vi "Slide Buttons.vi"(8 "error in (no error)":errorcluster, 10 "Distance":i32, 11 "Display State In":T1={"Numeric"=0.0, "Array of Button References"=[], "Space Between Menu Buttons"=0, "Number of Menu Buttons"=0, "Array of Button Names"=[], "Most Recent Vertical Position"=0, "This VI"=refnum, "Current Action"=enum."Not Moving", "Most Recent Distance Traveled"=0, "Method"=enum."Move Up", "Data In"=0} caption="State") -> (0 "error out":errorcluster, 3 "Display State Out":T1={"Numeric"=0.0, "Array of Button References"=[], "Space Between Menu Buttons"=0, "Number of Menu Buttons"=0, "Array of Button Names"=[], "Most Recent Vertical Position"=0, "This VI"=refnum, "Current Action"=enum."Not Moving", "Most Recent Distance Traveled"=0, "Method"=enum."Move Up", "Data In"=0} caption="State")   [LabVIEW 2011, in "Sliding Menu Library.lvlib" / "Sliding Menu XControl.xctl"]
uses:
  Sliding Menu xControl/Sliding Menu XControl.xctl
  Sliding Menu xControl/Sliding Menu State.ctl
  Menu Button Library/Menu Button xControl/Menu Button xControl.xctl
  Sliding Menu Type Definitions/Current User Action.ctl
  Sliding Menu xControl/Sliding Menu Methods.ctl
  Sliding Menu xControl/Sliding Menu Data.ctl
  Sliding Menu Library.lvlib
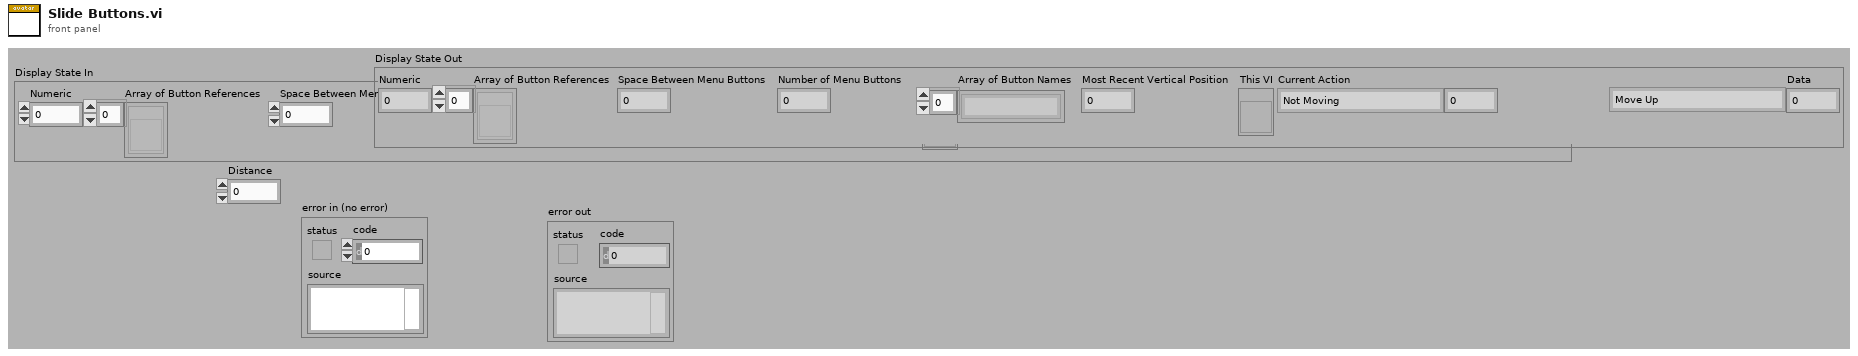
[diagram p1: front panel]
types:
  T1 = typedef "Sliding Menu Library.lvlib/Sliding Menu XControl.xctl/Sliding Menu State.ctl" = cluster{"Numeric":dbl, "Array of Button References":refnum<vi>[], "Space Between Menu Buttons":i32, "Number of Menu Buttons":i32, "Array of Button Names":string[], "Most Recent Vertical Position":i32, "This VI":refnum<vi>, "Current Action":T2, "Most Recent Distance Traveled":i32, "Method":T3, "Data In":T4}
  T2 = typedef "Sliding Menu Library.lvlib/Current User Action.ctl" = enum16{"Not Moving", "Mouse Down", "Mouse Up No Dragging", "Bounce Up Needed", "Bounce Down Needed", "Dragging", "Easing"}
  T3 = typedef "Sliding Menu Methods.ctl" = enum16{"Resize", "Move Up", "Move Down", "Move to 0"}
  T4 = typedef "Sliding Menu Library.lvlib/Sliding Menu XControl.xctl/Sliding Menu Data.ctl" = i32
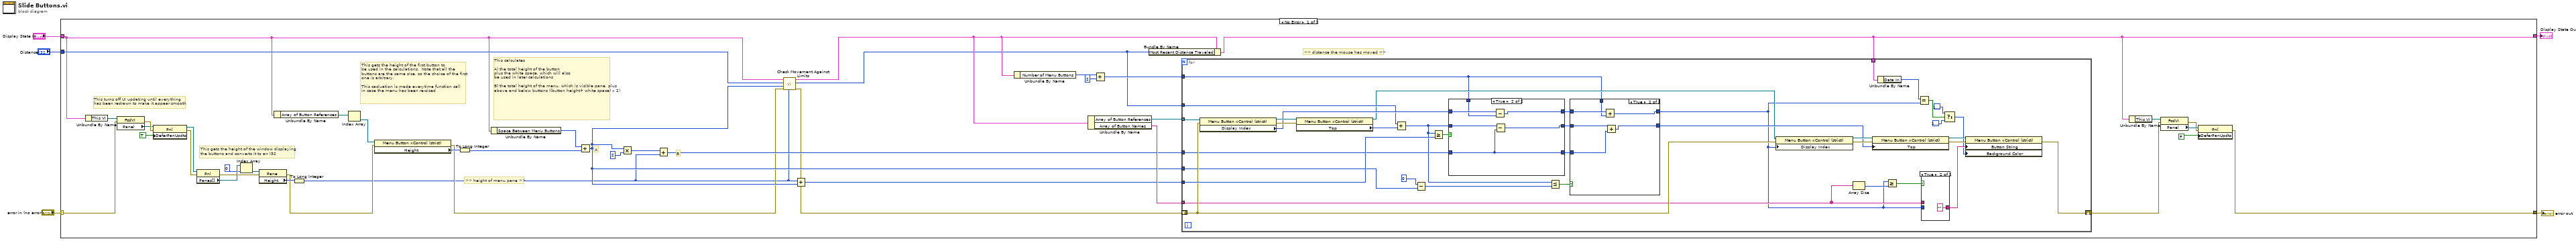
[diagram p0: block diagram]
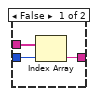
[diagram p2: hidden frame]
diagram:
  n1 = case shown="No Error" "error in (no error)" {
    selector: "error in (no error)" -> [w35 w107]
    tunnel: [w36 w107] -> w5
    tunnel: "Distance" -> [w14 _]
    tunnel: "Display State In" -> [w10 w106]
    tunnel: [w6 w106] -> w1
    frame No Error {
      # "B"
      # "A"
      # "This calculates \n\nA) the total height of the button\nplus the white space, which will also\nbe used in later calculations\n\nB) the total height of the menu, which is visible pane, plus above and below buttons ((button height+ white space) x 2)"
      # "This gets the height of the first button to \nbe used in the calculations.  Note that all the \nbuttons are the same size, so the choice of the first\none is arbitrary. \n\nThis cacluation is made everytime function call\nin case the menu has been re-sized"
      # "This gets the height of the window displaying\nthe buttons and converts it to an I32"
      # "This turns off UI updating until everything\nhas been redrawn to make it appear smooth"
      # ">> distance the mouse has moved >>"
      # ">> height of menu pane >>"
      n2 = Unbundle By Name(w10) -> ("This VI"=w47:refnum<vi>)
      n3 = property class="FcdVI"(reference=w47, error in=w35) -> (error out=w46:errorcluster, "Panel"=w45:refnum<vi>)  [unwired: 1 out]
      n4 = property class="Pnl"(reference=w45, error in=w46, "DeferPanUpdts"=TRUE ("Defer Panel Updates")) -> (reference out=w37:refnum<vi>, error out=w39:errorcluster)
      n5 = property class="Pnl"(reference=w37, error in=w39) -> (error out=w41:errorcluster, "Panes[]"=w43:refnum<vi>[])  [unwired: 1 out]
      n6 = Index Array(array=w43, index=0) -> (element=w40:refnum<vi>)
      n7 = property class="Pane"(reference=w40, error in=w41) -> (error out=w17:errorcluster, "Height"=w29:u32)  [unwired: 1 out]
      n8 = Unbundle By Name(w10) -> ("Array of Button References"=w33:refnum<vi>[])
      n9 = To Long Integer(number=w29) -> (32bit integer=w7:i32)
      n10 = Index Array(array=w33) -> (element=w34:refnum<vi>)  [unwired: 1 in]
      n11 = property class="Menu Button xControl (strict)"(reference=w34, error in=w17) -> (error out=w12:errorcluster, "Height"=w32:u32)  [unwired: 1 out]
      n12 = To Long Integer(number=w32) -> (32bit integer=w28:i32)
      n13 = Unbundle By Name(w10) -> ("Space Between Menu Buttons"=w19:i32)
      n14 = Add(x=w19, y=w28) -> (x+y=w13:i32)
      n15 = Multiply(x=w13, y=2) -> (x*y=w16:i32)
      n16 = Add(x=w16, y=w7) -> (x+y=w15:i32)
      n17 = call "Check Movement Against Limits.vi"("Height of Menu Pane"=w7, "error in"=w12, "Maximum Distance Away From Sides"=w13, "Distance Mouse Moved"=w14, "Display State In"=w10) -> ("error out"=w11:errorcluster, "Distance to Move"=w8:i32, "Display State In Out"=w9:T1)  [unwired: 4 in]
      n18 = Add(x=w7, y=w13) -> (x+y=w18:i32)
      n19 = Unbundle By Name(w9) -> ("Number of Menu Buttons"=w30:i32)
      n20 = Unbundle By Name(w9) -> ("Array of Button References"=w23:refnum<vi>[], "Array of Button Names"=w20:string[])
      n21 = Add(x=w30, y=2) -> (x+y=w21:i32)
      n22 = Bundle By Name(cluster=w9, "Most Recent Distance Traveled"=w8) -> (w6:T1)
      n23 = for {
        tunnel: w23 -> [w84] mode=indexing
        shift-right: [w65] -> w22
        shift-left: w11 -> [w66]
        tunnel: w21 -> [w60]
        tunnel: w8 -> [w71]
        tunnel: w20 -> [w58]
        tunnel: w18 -> [w76]
        tunnel: w13 -> [w61]
        tunnel: w15 -> [w55]
        tunnel: w6 -> [w54]
        n24 = property class="Menu Button xControl (strict)"(reference=w84, error in=w66) -> (reference out=w83:refnum<vi>, error out=w82:errorcluster, "Display Index"=w74:i32)
        n25 = property class="Menu Button xControl (strict)"(reference=w83, error in=w82) -> (reference out=w62:refnum<vi>, "Top"=w70:i32)  [unwired: 1 out]
        n26 = Add(x=w71, y=w70) -> (x+y=w69:i32)
        n27 = Subtract(x=0 ("y"), y=w61) -> (x-y=w63:i32)
        n28 = Greater Or Equal?(x=w69, y=w76) -> (x >= y?=w75:bool)
        n29 = case shown="True" w75 {
          tunnel: w74 -> [w99 w105]
          tunnel: [w99 w103] -> w72
          tunnel: w69 -> [w98 w102]
          tunnel: [w98 w101] -> w68
          tunnel: w60 -> [_ w104]
          tunnel: w55 -> [w97 w100]
          tunnel: [w97 w100] -> w59
          frame False {
          }
          frame True {
            n30 = Subtract(x=w105, y=w104) -> (x-y=w103:i32)
            n31 = Subtract(x=w102, y=w100) -> (x-y=w101:i32)
          }
        }
        n32 = Less Or Equal?(x=w69, y=w63) -> (x <= y?=w73:bool)
        n33 = case shown="True" w73 {
          tunnel: w72 -> [w90 w94]
          tunnel: [w90 w95] -> w52
          tunnel: [w89 w96] -> w67
          tunnel: w68 -> [w89 w93]
          tunnel: w60 -> [_ w92]
          tunnel: w59 -> [_ w91]
          frame False {
          }
          frame True {
            n34 = Add(x=w94, y=w92) -> (x+y=w95:i32)
            n35 = Add(x=w93, y=w91) -> (x+y=w96:i32)
          }
        }
        n36 = property class="Menu Button xControl (strict)"(reference=w62, error in=w66, "Display Index"=w52) -> (reference out=w80:refnum<vi>, error out=w81:errorcluster)
        n37 = Array Size(array=w58) -> (size(s)=w57:i32)
        n38 = property class="Menu Button xControl (strict)"(reference=w80, error in=w81, "Top"=w67) -> (reference out=w77:refnum<vi>, error out=w78:errorcluster)
        n39 = Unbundle By Name(w54) -> ("Data In"=w53:T4)
        n40 = Greater Or Equal?(x=w52, y=w57) -> (x >= y?=w56:bool)
        n41 = Equal?(x=w53, y=w52) -> (x = y?=w51:bool)
        n42 = case shown="True" w56 {
          tunnel: [w87 "" ("String")] -> w79
          tunnel: w58 -> [w86 _]
          tunnel: w52 -> [w85 _]
          frame False {
            n43 = Index Array(array=w86, index=w85) -> (element=w87:string)
          }
          frame True {
          }
        }
        n44 = Select(t=u32 16777238, s=w51, f=u32 16777216) -> (s? t:f=w48:u32)
        n45 = property class="Menu Button xControl (strict)"(reference=w77, error in=w78, "Button String"=w79, "Background Color"=w48) -> (error out=w65:errorcluster)  [unwired: 1 out]
      }
      n46 = Unbundle By Name(w6) -> ("This VI"=w26:refnum<vi>)
      n47 = property class="FcdVI"(reference=w26, error in=w22) -> (error out=w24:errorcluster, "Panel"=w25:refnum<vi>)  [unwired: 1 out]
      n48 = property class="Pnl"(reference=w25, error in=w24, "DeferPanUpdts"=FALSE ("Defer Panel Updates")) -> (error out=w36:errorcluster)  [unwired: 1 out]
    }
    frame Error {
    }
  }
  "error out" <- w5
  "Display State Out" <- w1
